vi "QA-Init Target VI.vi"(7 "error in (no error)":errorcluster, 10 "VI Refnum":refnum<vi>) -> (0 "error out":errorcluster, 3 "VI Refnum out":refnum<vi>)   [LabVIEW 2015]
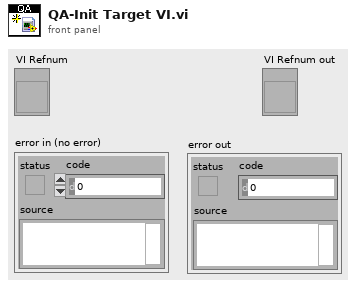
[diagram p1: front panel]
types:
  T1 = enum32{"Bad", "Idle", "Run top level", "Running"}
  T2 = enum32{"Invalid", "Standard", "Closed", "Hidden", "Minimized", "Maximized"}
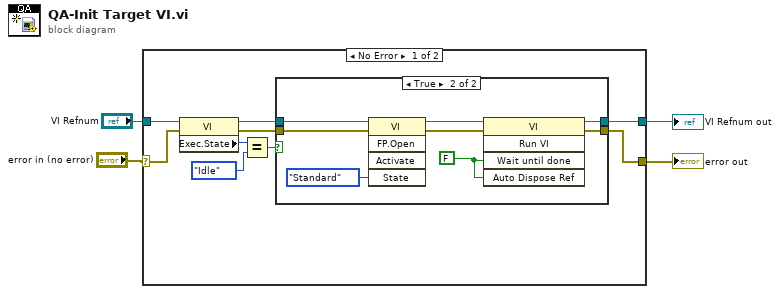
[diagram p0: block diagram]
diagram:
  n1 = case shown="No Error" "error in (no error)" {
    selector: "error in (no error)" -> [w5 w25]
    tunnel: [w13 w24] -> w4
    tunnel: "VI Refnum" -> [w10 w24]
    tunnel: [w9 w25] -> w2
    frame No Error {
      n2 = property class="VI"(reference=w10, error in=w5) -> (reference out=w6:refnum<vi>, error out=w7:errorcluster, "Exec.State"=w11:T1)
      n3 = Equal?(x=w11, y=T1."Idle" ("Execution:State")) -> (x = y?=w8:bool)
      n4 = case shown="True" w8 {
        tunnel: w6 -> [w15 w22]
        tunnel: w7 -> [w14 w21]
        tunnel: [w15 w20] -> w13
        tunnel: [w14 w19] -> w9
        frame False {
        }
        frame True {
          w23 = FALSE ("Wait Until Done")
          n5 = invoke class="VI" method="FP.Open"(reference=w22, error in=w21, "State"=T2."Standard") -> (reference out=w17:refnum<vi>, error out=w16:errorcluster)  [unwired: 2 in, 3 out]
          n6 = invoke class="VI" method="Run VI"(reference=w17, error in=w16, "Wait until done"=w23, "Auto Dispose Ref"=w23) -> (reference out=w20:refnum<vi>, error out=w19:errorcluster)  [unwired: 1 in, 3 out]
        }
      }
    }
    frame Error {
    }
  }
  "VI Refnum out" <- w4
  "error out" <- w2
